vi "Empty Rings.vi"(8 "error in (no error)":errorcluster, 11 "Ring References":refnum<vi>[](array[refnum])) -> (0 "error out":errorcluster, 3 "Array":refnum<vi>[](array[refnum]))   [LabVIEW 2019, in "Control Experiment.lvclass"]
uses:
  <userlib>/LevyLab/Transport/Control Experiment/Control Experiment.lvclass
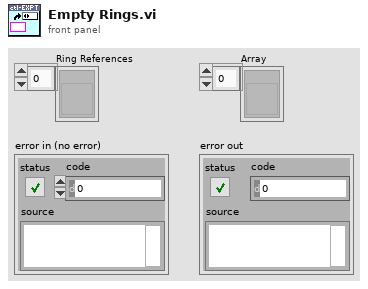
[diagram p1: front panel]
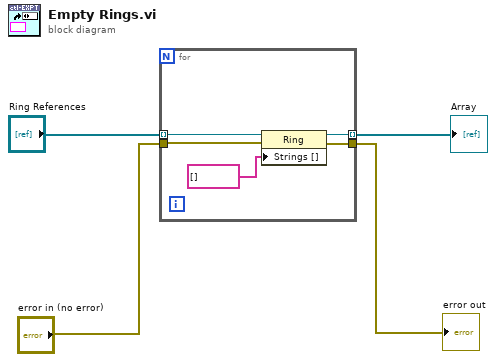
[diagram p0: block diagram]
diagram:
  n1 = for {
    tunnel: "Ring References" -> [w8] mode=indexing
    tunnel: "error in (no error)" -> [w7]
    tunnel: [w6] -> w1
    tunnel: [w5] -> w3 mode=indexing
    n2 = property class="Ring"(reference=w8, error in=w7, "Strings []"=string[] []) -> (reference out=w5:refnum<vi>, error out=w6:errorcluster)
  }
  "Array" <- w3
  "error out" <- w1
